vi "Get Output Terminals.vi"(9 "terminals datatypes":string[][](array[string]), 10 "isSource?":bool[](array[boolean]), 11 "isConnected?":bool[](array[boolean])) -> (3 "output terminals indexes":i32[](array[numeric]))   [LabVIEW 2014]
doc: "Returns indexes of output terminals stored in cluster."
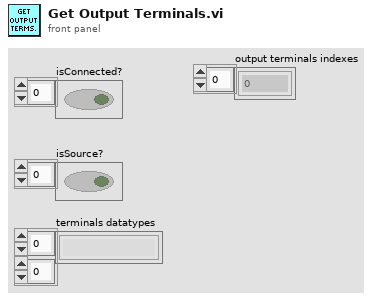
[diagram p1: front panel]
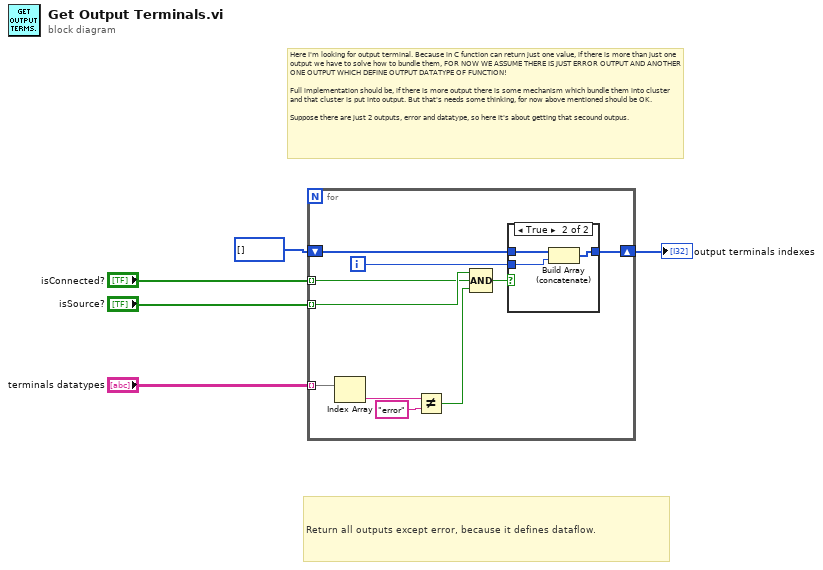
[diagram p0: block diagram]
diagram:
  # "Return all outputs except error, because it defines dataflow."
  # "Here I'm looking for output terminal. Because in C function can return just one value, if there is more than just one output we have to solve how to bundle them, FOR NOW WE ASSUME THERE IS JUST ERROR OUTPUT AND ANOTHER ONE OUTPUT WHICH DEFINE OUTPUT DATATYPE OF FUNCTION!\n\nFull implementation should be, if there is more output there is some mechanism which bundle them into cluster and that cluster is put into output. But that's needs some thinking, for now above mentioned should be OK.\n\nSuppose there are just 2 outputs, error and datatype, so here it's about getting that secound outpus."
  n1 = for {
    tunnel: "isSource?" -> [w14] mode=indexing
    tunnel: "isConnected?" -> [w13] mode=indexing
    tunnel: "terminals datatypes" -> [w12] mode=indexing
    shift-right: [w9] -> w5
    shift-left: i32[] [] -> [w10]
    i -> [w6]
    n2 = Index Array(array=w12) -> (element=w7:string)  [unwired: 1 in]
    n3 = Not Equal?(x=w7, y="error") -> (x != y?=w8:bool)
    n4 = Compound Arithmetic op=AND(w14, w13, w8) -> (w11:bool)
    n5 = case shown="True" w11 {
      tunnel: w6 -> [_ w17]
      tunnel: w10 -> [w16 w19]
      tunnel: [w16 w18] -> w9
      frame False {
      }
      frame True {
        n6 = Build Array (concatenate)(w19, w17) -> (w18:i32[])
      }
    }
  }
  "output terminals indexes" <- w5
